vi "subVI_getLightAttributes.vi"(11 "Cluster":T1) -> (0 "min_mireds":i32, 1 "max_mireds":i32, 2 "color_temp":i32, 3 "brightness":i32, 4 "state":bool)   [LabVIEW 2018]
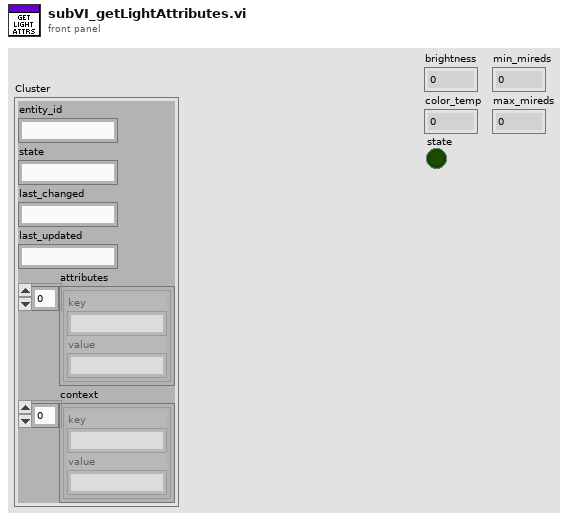
[diagram p1: front panel]
types:
  T1 = cluster{"entity_id":string, "state":string, "last_changed":string, "last_updated":string, "attributes":cluster{"key":string, "value":string}[], "context":cluster{"key":string, "value":string}[]}
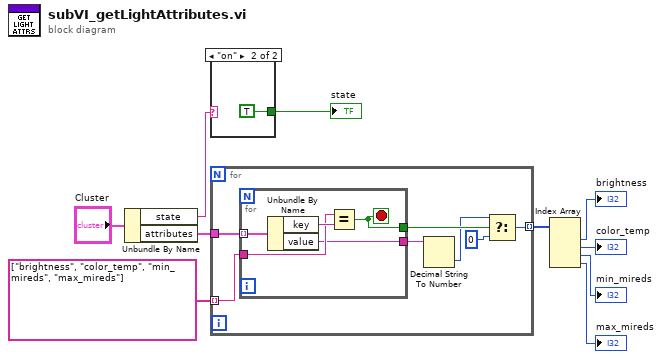
[diagram p0: block diagram]
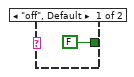
[diagram p2: hidden frame]
diagram:
  n1 = Unbundle By Name("Cluster") -> ("state"=w10:string, "attributes"=w8:cluster{"key":string, "value":string}[])
  n2 = case shown="\"on\"" w10 {
    tunnel: [FALSE TRUE] -> w1
    frame "off", Default {
    }
    frame "on" {
    }
  }
  "state" <- w1
  n3 = for {
    tunnel: w8 -> [w19]
    tunnel: string[] ["brightness", "color_temp", "min_mireds", "max_mireds"] -> [w14] mode=indexing
    tunnel: [w13] -> w6 mode=indexing
    n4 = for {
      tunnel: w19 -> [w24] mode=indexing
      tunnel: w14 -> [w22]
      tunnel: [w21] -> w15
      tunnel: [w20] -> w18
      stop <- w20 stop-if-true
      n5 = Unbundle By Name(w24) -> ("key"=w23:string, "value"=w21:string)
      n6 = Equal?(x=w22, y=w23) -> (x = y?=w20:bool)
    }
    n7 = Decimal String To Number(string=w15) -> (number=w16:i32)  [unwired: 2 in, 1 out]
    n8 = Select(t=w16, s=w18, f=0) -> (s? t:f=w13:i32)
  }
  n9 = Index Array(array=w6) -> (element #1=→"brightness":i32, element #2=→"color_temp":i32, element #3=→"min_mireds":i32, element #4=→"max_mireds":i32)  [unwired: 4 in]
